vi "Write Anything.vi"(7 "Format String (%#_13g)":string="%#_13g", 8 "Error In":errorcluster, 9 "Section Name (Name of \"Anything\")":string, 10 "Anything":variant, 11 "Path (dialog)":path) -> (0 "Error Out":errorcluster)   [LabVIEW 2012]
doc: "This VI is designed to write any data type to an INI file in human readable form. It will overwrite any data in the specified section of the INI file but leave other sections unchanged.\n\nFreeware from Moore Good Ideas, www.mooregoodideas.com. Do not remove this line."
uses:
  <vilib>/Utility/VariantDataType/VariantType.lvlib
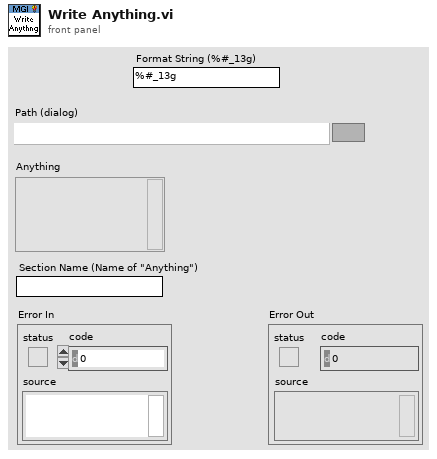
[diagram p1: front panel]
types:
  T1 = typedef "VariantType.lvlib/Type.ctl" = enum8{"Invalid Type", "Void", "I8", "I16", "I32", "I64", "U8", "U16", "U32", "U64", "Single Float", "Double Float", "Extended Float", "Single Complex", "Double Complex", "Extended Complex", "Enum U8", "Enum U16", "Enum U32", "Enum U64", "Single Float With Unit", "Double Float With Unit", "Extended Float With Unit", "Single Complex with Unit", "Double Complex with Unit", "Extended Complex with Unit", "Boolean", "String", "Path", "Picture", "Tag", "Array", "Cluster", "Variant", "LV Variant", "Waveform", "Timestamp", "Digital Waveform", "Digital Data", "ExpressData", "Refnum", "External Data", "VI", "Poly VI", "LabVIEW Class Instance", "Fixed Point"}
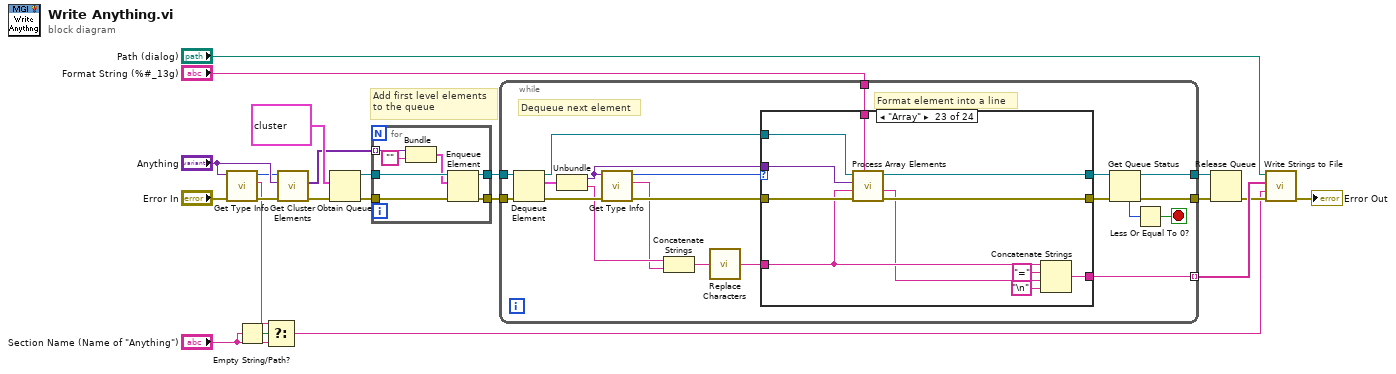
[diagram p0: block diagram]
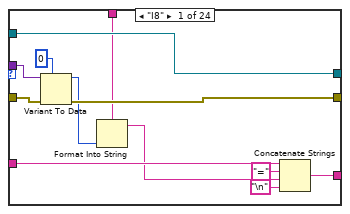
[diagram p2: hidden frame]
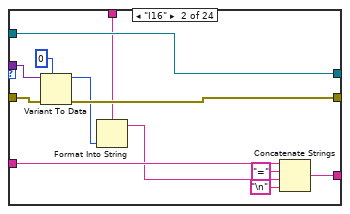
[diagram p3: hidden frame]
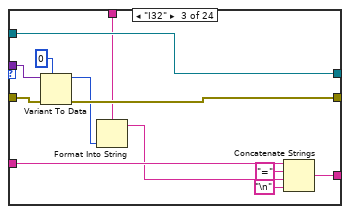
[diagram p4: hidden frame]
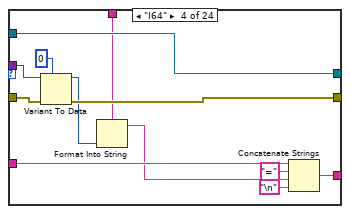
[diagram p5: hidden frame]
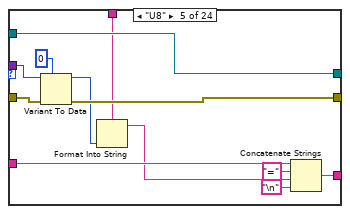
[diagram p6: hidden frame]
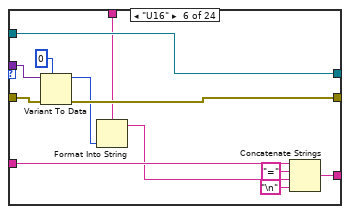
[diagram p7: hidden frame]
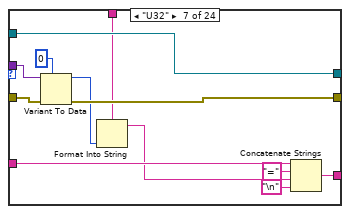
[diagram p8: hidden frame]
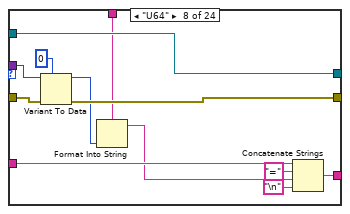
[diagram p9: hidden frame]
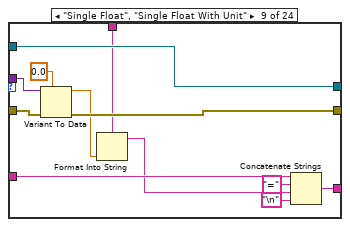
[diagram p10: hidden frame]
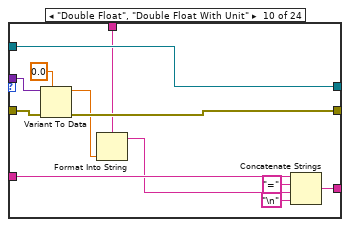
[diagram p11: hidden frame]
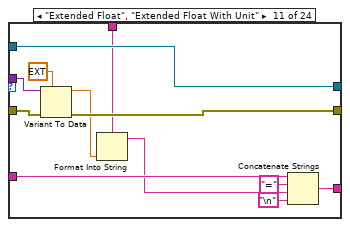
[diagram p12: hidden frame]
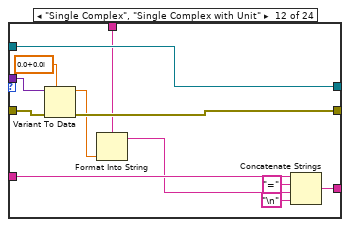
[diagram p13: hidden frame]
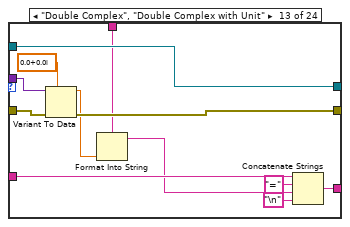
[diagram p14: hidden frame]
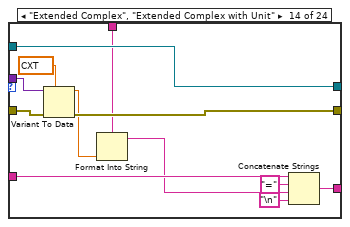
[diagram p15: hidden frame]
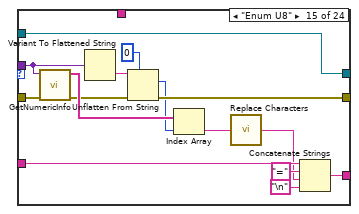
[diagram p16: hidden frame]
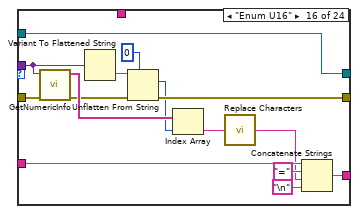
[diagram p17: hidden frame]
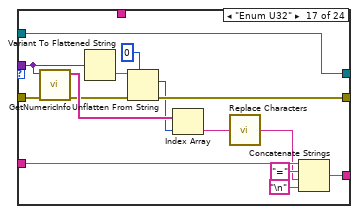
[diagram p18: hidden frame]
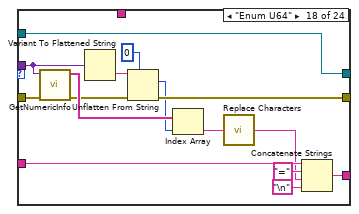
[diagram p19: hidden frame]
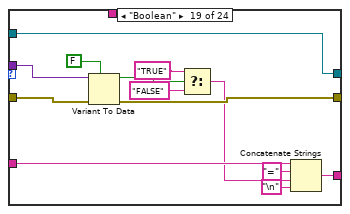
[diagram p20: hidden frame]
diagram:
  # "Add first level elements\nto the queue"
  n1 = call "Get Type Info.vi"("Error In"="Error In", "Variant"="Anything") -> ("Error Out"=w13:errorcluster, "Name"=w3:string, "Type Enum"=w6:T1)  [unwired: 7 in]
  n2 = Empty String/Path?(string/path="Section Name (Name of \"Anything\")") -> (empty?=w4:bool)
  n3 = Select(t=w3, s=w4, f="Section Name (Name of \"Anything\")") -> (s? t:f=w1:string)
  n4 = call "Get Cluster Elements.vi"("Error In"=w13, "Cluster"="Anything", "Type Enum (Cluster)"=w6) -> ("Error Out"=w10:errorcluster, "Cluster Elements"=w11:variant[])  [unwired: 7 in]
  n5 = Obtain Queue(element data type=cluster{"Variant":variant, "Name":string} {"Variant"=variant, "Name"=""}, error in (no error)=w10) -> (queue out=w21:refnum<queue>, error out=w20:errorcluster)  [unwired: 3 in, 1 out]
  n6 = for {
    tunnel: w21 -> [w29]
    tunnel: w20 -> [w28]
    tunnel: [w27] -> w19
    tunnel: [w26] -> w18
    tunnel: w11 -> [w24] mode=indexing
    n7 = Bundle("Variant"=w24, "") -> (w25:cluster{"Variant":variant, string})  [unwired: 1 in]
    n8 = Enqueue Element(queue=w29, element=w25, error in (no error)=w28) -> (queue out=w26:refnum<queue>, error out=w27:errorcluster)  [unwired: 1 in, 1 out]
  }
  n9 = while {
    tunnel: w19 -> [w49]
    tunnel: [w46] -> w17
    tunnel: [w34] -> w22 mode=indexing
    tunnel: w18 -> [w47]
    tunnel: [w43] -> w16
    tunnel: "Format String (%#_13g)" -> [w30]
    stop <- w44 stop-if-true
    # "Format element into a line"
    # "Dequeue next element"
    n10 = Dequeue Element(queue=w47, error in (no error)=w49) -> (queue out=w40:refnum<queue>, element=w38:cluster{"Variant":variant, "Name":string}, error out=w48:errorcluster)  [unwired: 1 in, 1 out]
    n11 = Unbundle(w38) -> ("Variant"=w37:variant, "Name"=w36:string)
    n12 = call "Get Type Info.vi"("Error In"=w48, "Variant"=w37) -> ("Error Out"=w35:errorcluster, "Name"=w33:string, "Type Enum"=w42:T1)  [unwired: 7 in]
    n13 = Concatenate Strings(w36, w33) -> (w32:string)
    n14 = call "Replace Characters.vi"("String In"=w32) -> ("String Out"=w31:string)  [unwired: 1 in]
    n15 = case shown="\"Array\"" w42 {
      selector: w42 -> [_ _ _ _ _ _ _ _ _ _ _ _ _ _ _ _ _ _ _ _ _ w319 _ _]
      tunnel: [w61 w73 w85 w97 w109 w121 w133 w145 w157 w169 w181 w193 w205 w217 w232 w247 w262 w277 w290 w301 w313 w323 w339 w356] -> w41
      tunnel: w40 -> [w61 w73 w85 w97 w109 w121 w133 w145 w157 w169 w181 w193 w205 w217 w232 w247 w262 w277 w290 w301 w313 w324 w343 w356]
      tunnel: [w57 w69 w81 w93 w105 w117 w129 w141 w153 w165 w177 w189 w201 w213 w226 w241 w256 w271 w289 w300 w312 w325 w340 w355] -> w39
      tunnel: w35 -> [w60 w72 w84 w96 w108 w120 w132 w144 w156 w168 w180 w192 w204 w216 w231 w246 w261 w276 w286 w297 w309 w321 w341 w355]
      tunnel: w31 -> [w54 w65 w77 w89 w101 w113 w125 w137 w149 w161 w173 w184 w196 w208 w220 w235 w250 w265 w279 w293 w304 w315 w335 w345]
      tunnel: w37 -> [w59 w71 w83 w95 w107 w119 w131 w143 w155 w167 w179 w191 w203 w215 w229 w244 w259 w274 w287 w298 w310 w318 w342 w354]
      tunnel: [w53 w66 w78 w90 w102 w114 w126 w138 w150 w162 w174 w185 w197 w209 w221 w236 w251 w266 w280 w294 w305 _ w336 w346] -> w34
      tunnel: w30 -> [w50 w62 w74 w88 w98 w110 w122 w134 w146 w159 w170 w182 w194 w206 _ _ _ _ _ _ _ _ w333 _]
      frame "I8" {
        n16 = Variant To Data(error in=w60, type=i8 0, Variant=w59) -> (data=w52:i8, error out=w57:errorcluster)
        n17 = Format Into String(format string=w50, w52) -> (resulting string=w51:string)  [unwired: 2 in, 1 out]
        n18 = Concatenate Strings(w54, "=" ("string"), w51, "\n") -> (w53:string)
      }
      frame "I16" {
        n19 = Variant To Data(error in=w72, type=i16 0, Variant=w71) -> (data=w63:i16, error out=w69:errorcluster)
        n20 = Format Into String(format string=w62, w63) -> (resulting string=w64:string)  [unwired: 2 in, 1 out]
        n21 = Concatenate Strings(w65, "=" ("string"), w64, "\n") -> (w66:string)
      }
      frame "I32" {
        n22 = Variant To Data(error in=w84, type=0, Variant=w83) -> (data=w76:i32, error out=w81:errorcluster)
        n23 = Format Into String(format string=w74, w76) -> (resulting string=w75:string)  [unwired: 2 in, 1 out]
        n24 = Concatenate Strings(w77, "=" ("string"), w75, "\n") -> (w78:string)
      }
      frame "I64" {
        n25 = Variant To Data(error in=w96, type=i64 0, Variant=w95) -> (data=w87:i64, error out=w93:errorcluster)
        n26 = Format Into String(format string=w88, w87) -> (resulting string=w86:string)  [unwired: 2 in, 1 out]
        n27 = Concatenate Strings(w89, "=" ("string"), w86, "\n") -> (w90:string)
      }
      frame "U8" {
        n28 = Variant To Data(error in=w108, type=u8 0, Variant=w107) -> (data=w100:u8, error out=w105:errorcluster)
        n29 = Format Into String(format string=w98, w100) -> (resulting string=w99:string)  [unwired: 2 in, 1 out]
        n30 = Concatenate Strings(w101, "=" ("string"), w99, "\n") -> (w102:string)
      }
      frame "U16" {
        n31 = Variant To Data(error in=w120, type=u16 0, Variant=w119) -> (data=w112:u16, error out=w117:errorcluster)
        n32 = Format Into String(format string=w110, w112) -> (resulting string=w111:string)  [unwired: 2 in, 1 out]
        n33 = Concatenate Strings(w113, "=" ("string"), w111, "\n") -> (w114:string)
      }
      frame "U32" {
        n34 = Variant To Data(error in=w132, type=u32 0, Variant=w131) -> (data=w124:u32, error out=w129:errorcluster)
        n35 = Format Into String(format string=w122, w124) -> (resulting string=w123:string)  [unwired: 2 in, 1 out]
        n36 = Concatenate Strings(w125, "=" ("string"), w123, "\n") -> (w126:string)
      }
      frame "U64" {
        n37 = Variant To Data(error in=w144, type=u64 0, Variant=w143) -> (data=w136:u64, error out=w141:errorcluster)
        n38 = Format Into String(format string=w134, w136) -> (resulting string=w135:string)  [unwired: 2 in, 1 out]
        n39 = Concatenate Strings(w137, "=" ("string"), w135, "\n") -> (w138:string)
      }
      frame "Single Float", "Single Float With Unit" {
        n40 = Variant To Data(error in=w156, type=sgl 0.0, Variant=w155) -> (data=w148:sgl, error out=w153:errorcluster)
        n41 = Format Into String(format string=w146, w148) -> (resulting string=w147:string)  [unwired: 2 in, 1 out]
        n42 = Concatenate Strings(w149, "=" ("string"), w147, "\n") -> (w150:string)
      }
      frame "Double Float", "Double Float With Unit" {
        n43 = Variant To Data(error in=w168, type=0.0, Variant=w167) -> (data=w160:dbl, error out=w165:errorcluster)
        n44 = Format Into String(format string=w159, w160) -> (resulting string=w158:string)  [unwired: 2 in, 1 out]
        n45 = Concatenate Strings(w161, "=" ("string"), w158, "\n") -> (w162:string)
      }
      frame "Extended Float", "Extended Float With Unit" {
        n46 = Variant To Data(error in=w180, type=ext 0.0, Variant=w179) -> (data=w172:ext, error out=w177:errorcluster)
        n47 = Format Into String(format string=w170, w172) -> (resulting string=w171:string)  [unwired: 2 in, 1 out]
        n48 = Concatenate Strings(w173, "=" ("string"), w171, "\n") -> (w174:string)
      }
      frame "Single Complex", "Single Complex with Unit" {
        n49 = Variant To Data(error in=w192, type=csg 0.0+0.0i, Variant=w191) -> (data=w188:csg, error out=w189:errorcluster)
        n50 = Format Into String(format string=w182, w188) -> (resulting string=w183:string)  [unwired: 2 in, 1 out]
        n51 = Concatenate Strings(w184, "=" ("string"), w183, "\n") -> (w185:string)
      }
      frame "Double Complex", "Double Complex with Unit" {
        n52 = Variant To Data(error in=w204, type=cdb 0.0+0.0i, Variant=w203) -> (data=w200:cdb, error out=w201:errorcluster)
        n53 = Format Into String(format string=w194, w200) -> (resulting string=w195:string)  [unwired: 2 in, 1 out]
        n54 = Concatenate Strings(w196, "=" ("string"), w195, "\n") -> (w197:string)
      }
      frame "Extended Complex", "Extended Complex with Unit" {
        n55 = Variant To Data(error in=w216, type=cxt 0.0+0.0i, Variant=w215) -> (data=w212:cxt, error out=w213:errorcluster)
        n56 = Format Into String(format string=w206, w212) -> (resulting string=w207:string)  [unwired: 2 in, 1 out]
        n57 = Concatenate Strings(w208, "=" ("string"), w207, "\n") -> (w209:string)
      }
      frame "Enum U8" {
        n58 = call <vilib>:"GetNumericInfo.vi"("error in (no error)"=w231, "Variant"=w229) -> ("error out"=w227:errorcluster, "EnumNames"=w230:string[])  [unwired: 6 in, 2 out]
        n59 = Variant To Flattened String(Variant=w229) -> (data string=w228:string)  [unwired: 1 out]
        n60 = Unflatten From String(type=u8 0, binary string=w228, error in (no error)=w227) -> (value=w225:u8, error out=w226:errorcluster)  [unwired: 2 in, 1 out]
        n61 = Index Array(array=w230, index=w225) -> (element=w219:string)
        n62 = call "Replace Characters.vi"("String In"=w219) -> ("String Out"=w218:string)  [unwired: 1 in]
        n63 = Concatenate Strings(w220, "=" ("string"), w218, "\n") -> (w221:string)
      }
      frame "Enum U16" {
        n64 = call <vilib>:"GetNumericInfo.vi"("error in (no error)"=w246, "Variant"=w244) -> ("error out"=w242:errorcluster, "EnumNames"=w245:string[])  [unwired: 6 in, 2 out]
        n65 = Variant To Flattened String(Variant=w244) -> (data string=w243:string)  [unwired: 1 out]
        n66 = Unflatten From String(type=u16 0, binary string=w243, error in (no error)=w242) -> (value=w240:u16, error out=w241:errorcluster)  [unwired: 2 in, 1 out]
        n67 = Index Array(array=w245, index=w240) -> (element=w234:string)
        n68 = call "Replace Characters.vi"("String In"=w234) -> ("String Out"=w233:string)  [unwired: 1 in]
        n69 = Concatenate Strings(w235, "=" ("string"), w233, "\n") -> (w236:string)
      }
      frame "Enum U32" {
        n70 = call <vilib>:"GetNumericInfo.vi"("error in (no error)"=w261, "Variant"=w259) -> ("error out"=w257:errorcluster, "EnumNames"=w260:string[])  [unwired: 6 in, 2 out]
        n71 = Variant To Flattened String(Variant=w259) -> (data string=w258:string)  [unwired: 1 out]
        n72 = Unflatten From String(type=u32 0, binary string=w258, error in (no error)=w257) -> (value=w255:u32, error out=w256:errorcluster)  [unwired: 2 in, 1 out]
        n73 = Index Array(array=w260, index=w255) -> (element=w249:string)
        n74 = call "Replace Characters.vi"("String In"=w249) -> ("String Out"=w248:string)  [unwired: 1 in]
        n75 = Concatenate Strings(w250, "=" ("string"), w248, "\n") -> (w251:string)
      }
      frame "Enum U64" {
        n76 = call <vilib>:"GetNumericInfo.vi"("error in (no error)"=w276, "Variant"=w274) -> ("error out"=w272:errorcluster, "EnumNames"=w275:string[])  [unwired: 6 in, 2 out]
        n77 = Variant To Flattened String(Variant=w274) -> (data string=w273:string)  [unwired: 1 out]
        n78 = Unflatten From String(type=u64 0, binary string=w273, error in (no error)=w272) -> (value=w270:u64, error out=w271:errorcluster)  [unwired: 2 in, 1 out]
        n79 = Index Array(array=w275, index=w270) -> (element=w264:string)
        n80 = call "Replace Characters.vi"("String In"=w264) -> ("String Out"=w263:string)  [unwired: 1 in]
        n81 = Concatenate Strings(w265, "=" ("string"), w263, "\n") -> (w266:string)
      }
      frame "Boolean" {
        n82 = Variant To Data(error in=w286, type=FALSE, Variant=w287) -> (data=w285:bool, error out=w289:errorcluster)
        n83 = Select(t="TRUE", s=w285, f="FALSE") -> (s? t:f=w278:string)
        n84 = Concatenate Strings(w279, "=" ("string"), w278, "\n") -> (w280:string)
      }
      frame "String" {
        n85 = Variant To Data(error in=w297, type="", Variant=w298) -> (data=w292:string, error out=w300:errorcluster)
        n86 = call "Replace Characters.vi"("String In"=w292) -> ("String Out"=w291:string)  [unwired: 1 in]
        n87 = Concatenate Strings(w293, "=" ("string"), w291, "\n") -> (w294:string)
      }
      frame "Path" {
        n88 = Variant To Data(error in=w309, type=path "", Variant=w310) -> (data=w308:path, error out=w312:errorcluster)
        n89 = Path To String(path=w308) -> (string=w303:string)
        n90 = call "Replace Characters.vi"("String In"=w303) -> ("String Out"=w302:string)  [unwired: 1 in]
        n91 = Concatenate Strings(w304, "=" ("string"), w302, "\n") -> (w305:string)
      }
      frame "Cluster" {
        # "Enqueue cluster elements"
        n92 = call "Get Cluster Elements.vi"("Error In"=w321, "Cluster"=w318, "Type Enum (Cluster)"=w319) -> ("Error Out"=w320:errorcluster, "Cluster Elements"=w317:variant[])  [unwired: 7 in]
        n93 = Concatenate Strings(w315, "." ("string")) -> (w314:string)
        n94 = Reverse 1D Array(array=w317) -> (reversed array=w322:variant[])
        n95 = for {
          tunnel: w324 -> [w332]
          tunnel: w320 -> [w331]
          tunnel: [w330] -> w325
          tunnel: [w329] -> w323
          tunnel: w322 -> [w327] mode=indexing
          tunnel: w314 -> [w326]
          n96 = Bundle("Variant"=w327, w326) -> (w328:cluster{"Variant":variant, string})  [unwired: 1 in]
          n97 = Enqueue Element At Opposite End(queue=w332, element=w328, error in (no error)=w331) -> (queue out=w329:refnum<queue>, error out=w330:errorcluster)  [unwired: 1 in, 1 out]
        }
      }
      frame "Array" {
        n98 = call "Process Array Elements.vi"("Format String (%#0.15f)"=w333, "Error In"=w341, "Name In"=w335, "Array Variant"=w342, "Queue In"=w343) -> ("Error Out"=w340:errorcluster, "Data Out"=w334:string, "Queue Out"=w339:refnum<queue>)  [unwired: 4 in]
        n99 = Concatenate Strings(w335, "=" ("string"), w334, "\n") -> (w336:string)
      }
      frame Default {
        n100 = Variant To Flattened String(Variant=w354) -> (data string=w349:string)  [unwired: 1 out]
        n101 = String To Byte Array(string=w349) -> (unsigned byte array=w353:u8[])
        n102 = Number To Hexadecimal String(1:i16 2 ("width (-)"), 2:w353) -> (0:w352:string[])
        n103 = Concatenate Strings("0x", w352) -> (w344:string)
        n104 = Concatenate Strings(w345, "=" ("string"), w344, "\n") -> (w346:string)
      }
    }
    n105 = Get Queue Status(queue=w41, error in (no error)=w39) -> (queue out=w43:refnum<queue>, error out=w46:errorcluster, # elements in queue=w45:i32)  [unwired: 1 in, 5 out]
    n106 = Less Or Equal To 0?(x=w45) -> (x <= 0?=w44:bool)
  }
  n107 = Release Queue(queue=w16, error in (no error)=w17) -> (error out=w8:errorcluster)  [unwired: 1 in, 2 out]
  n108 = call "Write Strings to File.vi"("Error In"=w8, "Section Name"=w1, "Array of Strings"=w22, "Path"="Path (dialog)") -> ("Error Out"=→"Error Out":errorcluster)  [unwired: 7 in]
